vi "LJM logger process new open.vi"(0 "Handle":i32, 5 "Device Type String":string, 7 "Connection Type String":string, 9 "Identifier String":string) -> (4 "Handle Out":i32, 8 "Opened Device Params":T1={"Device Type"="ANY", "Connection Type"="ANY", "Serial Number"=0}, 15 "error out":errorcluster)   [LabVIEW 2026]
uses:
  Common Logger Controls/Currently Opened Device Params.ctl
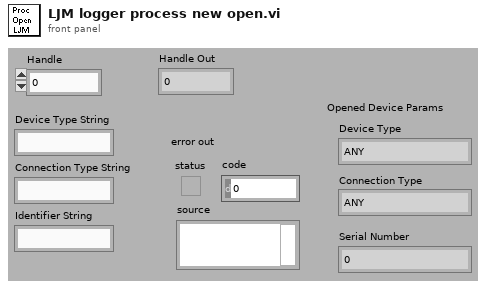
[diagram p1: front panel]
types:
  T1 = typedef "Currently Opened Device Params.ctl" = cluster{"Device Type":string, "Connection Type":string, "Serial Number":i32}
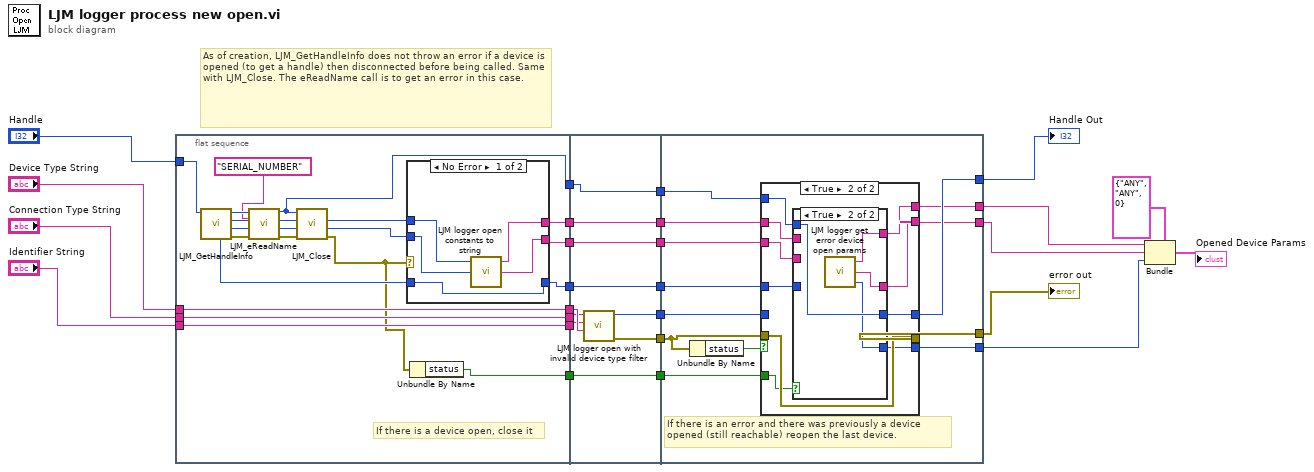
[diagram p0: block diagram]
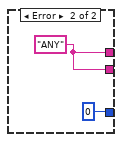
[diagram p2: hidden frame]
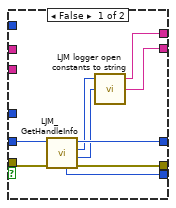
[diagram p3: hidden frame]
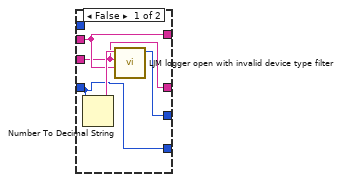
[diagram p4: hidden frame]
diagram:
  # "As of creation, LJM_GetHandleInfo does not throw an error if a device is opened (to get a handle) then disconnected before being called. Same with LJM_Close. The eReadName call is to get an error in this case."
  n1 = flat-sequence {
    tunnel: "Device Type String" -> [w41]
    tunnel: "Identifier String" -> [w42]
    tunnel: "Connection Type String" -> [w43]
    tunnel: [w43] -> w20
    tunnel: [w42] -> w19
    tunnel: [w41] -> w18
    tunnel: "Handle" -> [w32]
    tunnel: [w37] -> w17
    tunnel: [w36] -> w16
    tunnel: [w35] -> w15
    tunnel: [w34] -> w14
    tunnel: [w27] -> w13
    tunnel: w20 -> [w59]
    tunnel: w19 -> [w58]
    tunnel: w18 -> [w60]
    tunnel: [w57] -> w12
    tunnel: [w56] -> w11
    tunnel: [w55] -> w10
    tunnel: w17 -> [w55]
    tunnel: w16 -> [w54]
    tunnel: [w54] -> w9
    tunnel: [w53] -> w8
    tunnel: w15 -> [w53]
    tunnel: [w52] -> w7
    tunnel: w14 -> [w52]
    tunnel: w13 -> [w51]
    tunnel: [w51] -> w6
    tunnel: [w73] -> w22
    tunnel: [w72] -> w26
    tunnel: [w71] -> w3
    tunnel: w12 -> [w70]
    tunnel: w11 -> [w69]
    tunnel: [w68] -> w1
    tunnel: [w67] -> w2
    tunnel: w10 -> [w65]
    tunnel: w9 -> [w64]
    tunnel: w8 -> [w63]
    tunnel: w7 -> [w62]
    tunnel: w6 -> [w61]
    frame #0 {
      # "If there is a device open, close it"
      n2 = call "LJM_GetHandleInfo.vi"("Handle In"=w32) -> ("error out"=w30:errorcluster, "ConnectionType"=w39:i32, "DeviceType"=w38:i32, "Handle Out"=w31:i32, "SerialNumber"=w40:i32)  [unwired: 3 in, 3 out]
      n3 = call "LJM_eReadName.vi"("Handle In"=w31, "Name"="SERIAL_NUMBER", "error in"=w30) -> ("Handle Out"=w27:i32, "error out"=w29:errorcluster)  [unwired: 10 in, 1 out]
      n4 = call "LJM_Close.vi"("error in"=w29, "Handle"=w27) -> ("error out"=w33:errorcluster)  [unwired: 9 in]
      n5 = case shown="No Error" w33 {
        tunnel: w38 -> [w48 _]
        tunnel: w39 -> [w47 _]
        tunnel: [w46 w50] -> w37
        tunnel: [w45 w50] -> w36
        tunnel: w40 -> [w44 _]
        tunnel: [w44 0 ("SerialNumber")] -> w35
        frame No Error {
          n6 = call "LJM logger open constants to string.vi"("ConnType"=w47, "DevType"=w48) -> ("ConnTypeString"=w45:string, "DevTypeString"=w46:string)  [unwired: 2 in]
        }
        frame Error {
          w50 = "ANY" ("DevTypeString")
        }
      }
      n7 = Unbundle By Name(w33) -> ("status"=w34:bool)
    }
    frame #1 {
      n8 = call "LJM logger open with invalid device type filter.vi"("DeviceType"=w60, "ConnectionType"=w59, "Identifier"=w58) -> ("error out"=w57:errorcluster, "Handle"=w56:i32)  [unwired: 3 in]
    }
    frame #2 {
      # "If there is an error and there was previously a device \nopened (still reachable) reopen the last device."
      n9 = Unbundle By Name(w70) -> ("status"=w66:bool)
      n10 = case shown="True" w66 {
        tunnel: [w81 w91] -> w73
        tunnel: [w82 w92] -> w72
        tunnel: [w80 w83] -> w71
        tunnel: w70 -> [w79 w91]
        tunnel: w69 -> [w78 _]
        tunnel: [w75 w84] -> w68
        tunnel: [w74 w85] -> w67
        tunnel: w65 -> [_ w90]
        tunnel: w64 -> [_ w89]
        tunnel: w63 -> [_ w88]
        tunnel: w62 -> [_ w87]
        tunnel: w61 -> [_ w86]
        frame False {
          n11 = call "LJM_GetHandleInfo.vi"("error in"=w79, "Handle In"=w78) -> ("error out"=w81:errorcluster, "ConnectionType"=w76:i32, "DeviceType"=w77:i32, "Handle Out"=w82:i32, "SerialNumber"=w80:i32)  [unwired: 2 in, 3 out]
          n12 = call "LJM logger open constants to string.vi"("ConnType"=w76, "DevType"=w77) -> ("ConnTypeString"=w74:string, "DevTypeString"=w75:string)  [unwired: 2 in]
        }
        frame True {
          n13 = case shown="True" w87 {
            tunnel: [w96 w101] -> w92
            tunnel: w90 -> [w95 _]
            tunnel: w89 -> [w94 _]
            tunnel: w88 -> [w93 _]
            tunnel: w86 -> [_ w101]
            tunnel: [w95 w100] -> w84
            tunnel: [w94 w99] -> w85
            tunnel: [w93 w98] -> w83
            frame False {
              n14 = Number To Decimal String(number=w93) -> (decimal integer string=w97:string)  [unwired: 1 in]
              n15 = call "LJM logger open with invalid device type filter.vi"("DeviceType"=w95, "ConnectionType"=w94, "Identifier"=w97) -> ("Handle"=w96:i32)  [unwired: 3 in, 1 out]
            }
            frame True {
              n16 = call "LJM logger get error device open params.vi"() -> ("Serial Number"=w98:i32, "Connection Type"=w99:string, "Device Type"=w100:string)
            }
          }
        }
      }
    }
  }
  n17 = Bundle(cluster=T1 {"Device Type"="ANY", "Connection Type"="ANY", "Serial Number"=0} ("Current Device Connection"), "Device Type"=w1, "Connection Type"=w2, "Serial Number"=w3) -> (→"Opened Device Params":T1)
  "Handle Out" <- w26
  "error out" <- w22
